vi "Write Item HL.vi"(6 "itemName":string, 7 "Numeric":sgl, 8 "error in":errorcluster, 9 "AddItems":refnum<k24>[](array[refnum]), 10 "CreateSubscription in":refnum<k24>, 11 ".Server Refnum in":refnum<k24>) -> (0 "error out":errorcluster, 2 "Array":string[](array[string]), 3 ".NET Refnum out":refnum<k24>)   [LabVIEW 2024, in "LV_OPC_NET.lvlib"]
uses:
  LV_OPC_NET.lvlib
  C:/Users/Andrey/Desktop/LV_OPC-Client-x64/LV_OPC_Test/OPC.NET/OpcNetApi.dll
  OpcNetApi.dll
  System.Xml
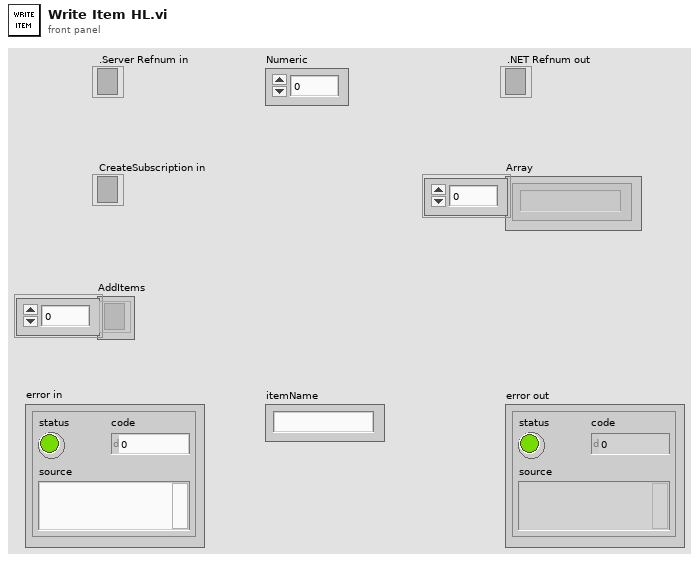
[diagram p1: front panel]
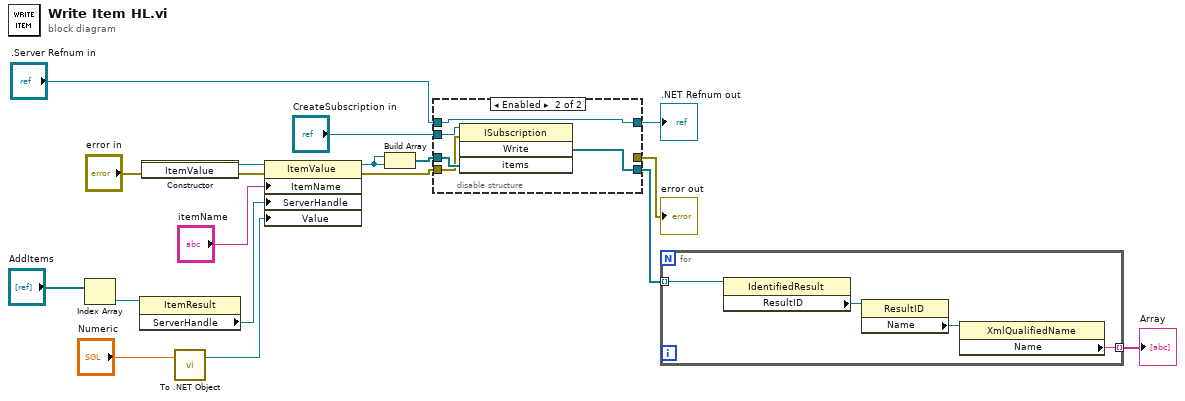
[diagram p0: block diagram]
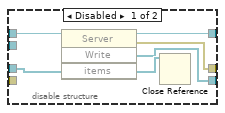
[diagram p2: hidden frame]
diagram:
  n1 = Index Array(array="AddItems") -> (element=w15:refnum<k24>)  [unwired: 1 in]
  n2 = property class="ItemResult"(reference=w15) -> ("ServerHandle"=w16:refnum<k24>)  [unwired: 1 in, 2 out]
  n3 = constructor class="ItemValue"(error in="error in") -> (reference out=w6:refnum<k24>, error out=w3:errorcluster)  [unwired: 2 in, 1 out]
  n4 = call <vilib>:"To .NET Object.vi"("anything"="Numeric") -> (".NET object"=w9:refnum<k24>)  [unwired: 1 in, 1 out]
  n5 = property class="ItemValue"(reference=w6, error in=w3, "ItemName"="itemName", "ServerHandle"=w16, "Value"=w9) -> (reference out=w1:refnum<k24>, error out=w2:errorcluster)
  n6 = Build Array(w1, w1) -> (w8:refnum<k24>[])
  n7 = disable-structure shown="Enabled" {
    disable-tunnel: [w24 _] -> w5
    disable-tunnel: [w23 w27] -> w7
    disable-tunnel: w8 -> [w22 w29]
    disable-tunnel: ".Server Refnum in" -> [w20 w27]
    disable-tunnel: "CreateSubscription in" -> [_ w28]
    disable-tunnel: [w19 w26] -> w12
    disable-tunnel: w2 -> [_ w25]
    frame Disabled {
      n8 = invoke class="Server" method="Write"(reference=w20, "items"=w22) -> (reference out=w23:refnum<k24>, error out=w24:errorcluster, "Write"=w19:refnum<k24>[], "items"=w21:refnum<k24>[])  [unwired: 2 in]
      n9 = Close Reference(reference=w21) -> ()  [unwired: 1 in, 1 out]
    }
    frame Enabled {
      n10 = invoke class="ISubscription" method="Write"(reference=w28, error in=w25, "items"=w29) -> ("Write"=w26:refnum<k24>[])  [unwired: 1 in, 3 out]
    }
  }
  ".NET Refnum out" <- w7
  "error out" <- w5
  n11 = for {
    tunnel: w12 -> [w33] mode=indexing
    tunnel: [w30] -> w13 mode=indexing
    n12 = property class="IdentifiedResult"(reference=w33) -> ("ResultID"=w32:refnum<k24>)  [unwired: 1 in, 2 out]
    n13 = property class="ResultID"(reference=w32) -> ("Name"=w31:refnum<k24>)  [unwired: 1 in, 2 out]
    n14 = property class="XmlQualifiedName"(reference=w31) -> ("Name"=w30:string)  [unwired: 1 in, 2 out]
  }
  "Array" <- w13
